vi "Pulser Fail Warning.vi"(0 "Pulser":T1=enum."Agilent 33xxx", 5 "Agilent":refnum<visa-resource-name>="COM8", 7 "JSR":refnum<visa-resource-name>="COM8", 9 "Panametrics":refnum<visa-resource-name>="COM8", 11 "UTEX":refnum<visa-resource-name>="COM8") -> (4 "Pulser Out":T1=enum."Agilent 33xxx", 6 "Agilent Out":refnum<visa-resource-name>, 8 "JSR Out":refnum<visa-resource-name>, 10 "Panametrics Out":refnum<visa-resource-name>, 14 "Retry":bool, 15 "UTEX Out":refnum<visa-resource-name>)   [LabVIEW 2022 SP3]
uses:
  pulser.ctl
panel:
  in  "Ignore":bool
  in  "Abort":bool
  in  "Try Again":bool
  # "Pulser Initialization Failed!"
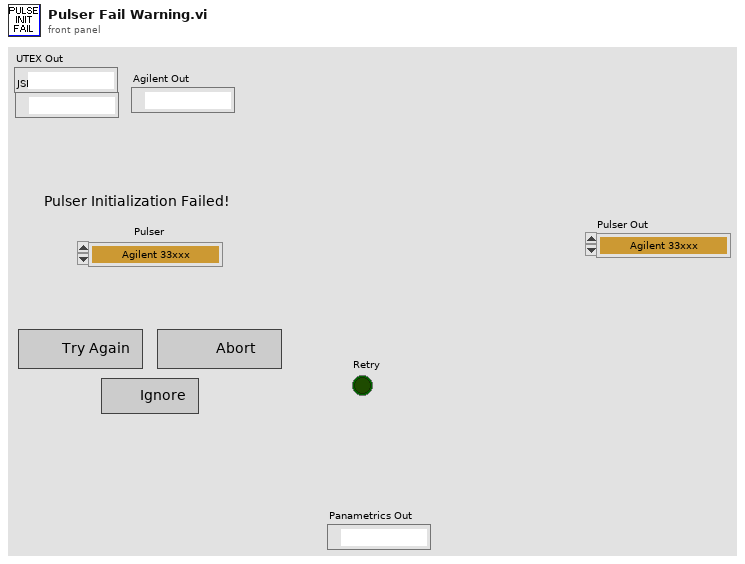
[diagram p1: front panel]
types:
  T1 = typedef "pulser.ctl" = enum16{"Pan 5900", "Daxsonics", "Agilent 33xxx", "UTEX", "JSR", "WMC Mono-Cycle", "No Pulser", "NYU AVTECH", "Tabor W1281A", "Pan 5800", "Unlisted", "Tabor WX2182B"}
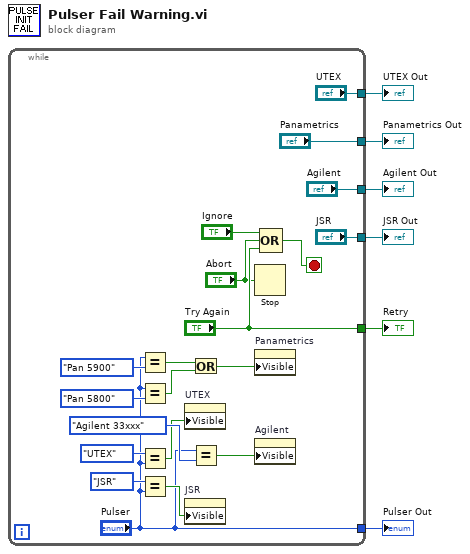
[diagram p0: block diagram]
diagram:
  n1 = while {
    tunnel: ["Pulser"] -> w5
    tunnel: ["Try Again"] -> w6
    tunnel: ["Agilent"] -> w4
    tunnel: ["Panametrics"] -> w3
    tunnel: ["JSR"] -> w2
    tunnel: ["UTEX"] -> w1
    stop <- w26 stop-if-true
    n2 = Equal?(x="Pulser", y=pulser."Pan 5900") -> (x = y?=w19:bool)
    n3 = Equal?(x="Pulser", y=pulser."Pan 5800") -> (x = y?=w17:bool)
    n4 = Equal?(x=pulser."UTEX" ("y"), y="Pulser") -> (x = y?=w7:bool)
    n5 = Equal?(x=pulser."JSR" ("y"), y="Pulser") -> (x = y?=w11:bool)
    n6 = property on="UTEX" class="VISAName"("Visible"=w7) -> ()  [unwired: 2 in, 2 out]
    n7 = property on="JSR" class="VISAName"("Visible"=w11) -> ()  [unwired: 2 in, 2 out]
    n8 = Or(x=w19, y=w17) -> (x .or. y?=w18:bool)
    n9 = Equal?(x="Pulser", y=pulser."Agilent 33xxx") -> (x = y?=w23:bool)
    n10 = Stop(stop? (T)="Abort") -> ()
    n11 = property on="Panametrics" class="VISAName"("Visible"=w18) -> ()  [unwired: 2 in, 2 out]
    n12 = property on="Agilent" class="VISAName"("Visible"=w23) -> ()  [unwired: 2 in, 2 out]
    n13 = Compound Arithmetic op=OR("Ignore", "Abort", "Try Again") -> (w26:bool)
  }
  "Pulser Out" <- w5
  "Retry" <- w6
  "Agilent Out" <- w4
  "Panametrics Out" <- w3
  "JSR Out" <- w2
  "UTEX Out" <- w1
